vi "Vision Processing Boulder.vi"(4 "error in (no error)":errorcluster) -> ()   [LabVIEW 2015]
doc: "This VI runs in parallel to other tasks. It gets images from the camera, processes them for color or shape and uses commands or globals to affect the behavior of other subsystems."
uses:
  Framework/Robot Global Data.vi
  Support Code/ZMQ Library/socket_options.ctl
  Support Code/ZMQ Library/zeromq.lvlib
  Support Code/ZMQ Library/socket_type.ctl
  Support Code/ZMQ Library/zmq_context.lvclass
  Support Code/ZMQ Library/zmq_socket.lvclass
  Vision Published Globals.vi
  Intake/Implementation/Intake Published Globals.vi
panel:
  out "context out":refnum<class "zmq_context.lvclass">
  out "data 2":string
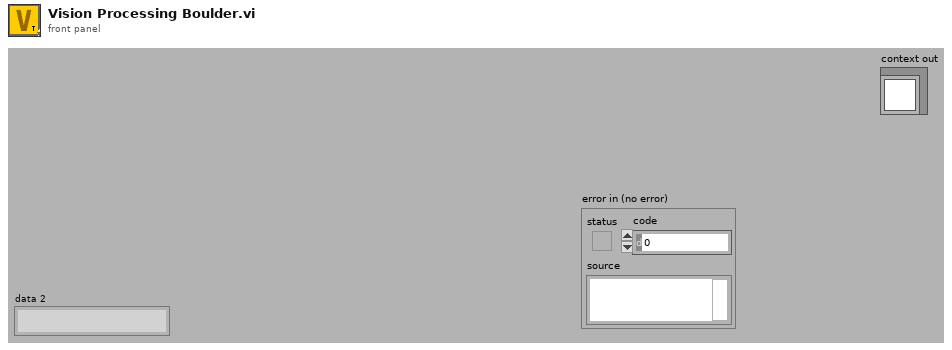
[diagram p1: front panel]
types:
  T1 = typedef "zeromq.lvlib/socket_options.ctl" = enum8{"NONE", "ZMQ_HWM", "<2>", "ZMQ_SWAP", "ZMQ_AFFINITY", "ZMQ_IDENTITY", "ZMQ_SUBSCRIBE", "ZMQ_UNSUBSCRIBE", "ZMQ_RATE", "ZMQ_RECOVERY_IVL", "ZMQ_MCAST_LOOP", "ZMQ_SNDBUF", "ZMQ_RCVBUF", "ZMQ_RCVMORE", "ZMQ_FD", "ZMQ_EVENTS", "ZMQ_TYPE", "ZMQ_LINGER", "ZMQ_RECONNECT_IVL", "ZMQ_BACKLOG", "ZMQ_RECOVERY_IVL_MSEC", "ZMQ_RECONNECT_IVL_MAX", "ZMQ_MAXMSGSIZE", "ZMQ_SNDHWM", "ZMQ_RCVHWM", "ZMQ_MULTICAST_HOPS", "<26>", "ZMQ_RCVTIMEO", "ZMQ_SNDTIMEO", "<29>", "<30>", "ZMQ_IPV4ONLY", "ZMQ_LAST_ENDPOINT", "ZMQ_ROUTER_MANDATORY", "ZMQ_TCP_KEEPALIVE", "ZMQ_TCP_KEEPALIVE_CNT", "ZMQ_TCP_KEEPALIVE_IDLE", "ZMQ_TCP_KEEPALIVE_INTVL", "ZMQ_TCP_ACCEPT_FILTER", "ZMQ_DELAY_ATTACH_ON_CONNECT", "ZMQ_XPUB_VERBOSE"}
  T2 = typedef "zeromq.lvlib/socket_type.ctl" = enum8{"ZMQ_PAIR", "ZMQ_PUB", "ZMQ_SUB", "ZMQ_REQ", "ZMQ_REP", "ZMQ_DEALER", "ZMQ_ROUTER", "ZMQ_PULL", "ZMQ_PUSH", "ZMQ_XPUB", "ZMQ_XSUB"}
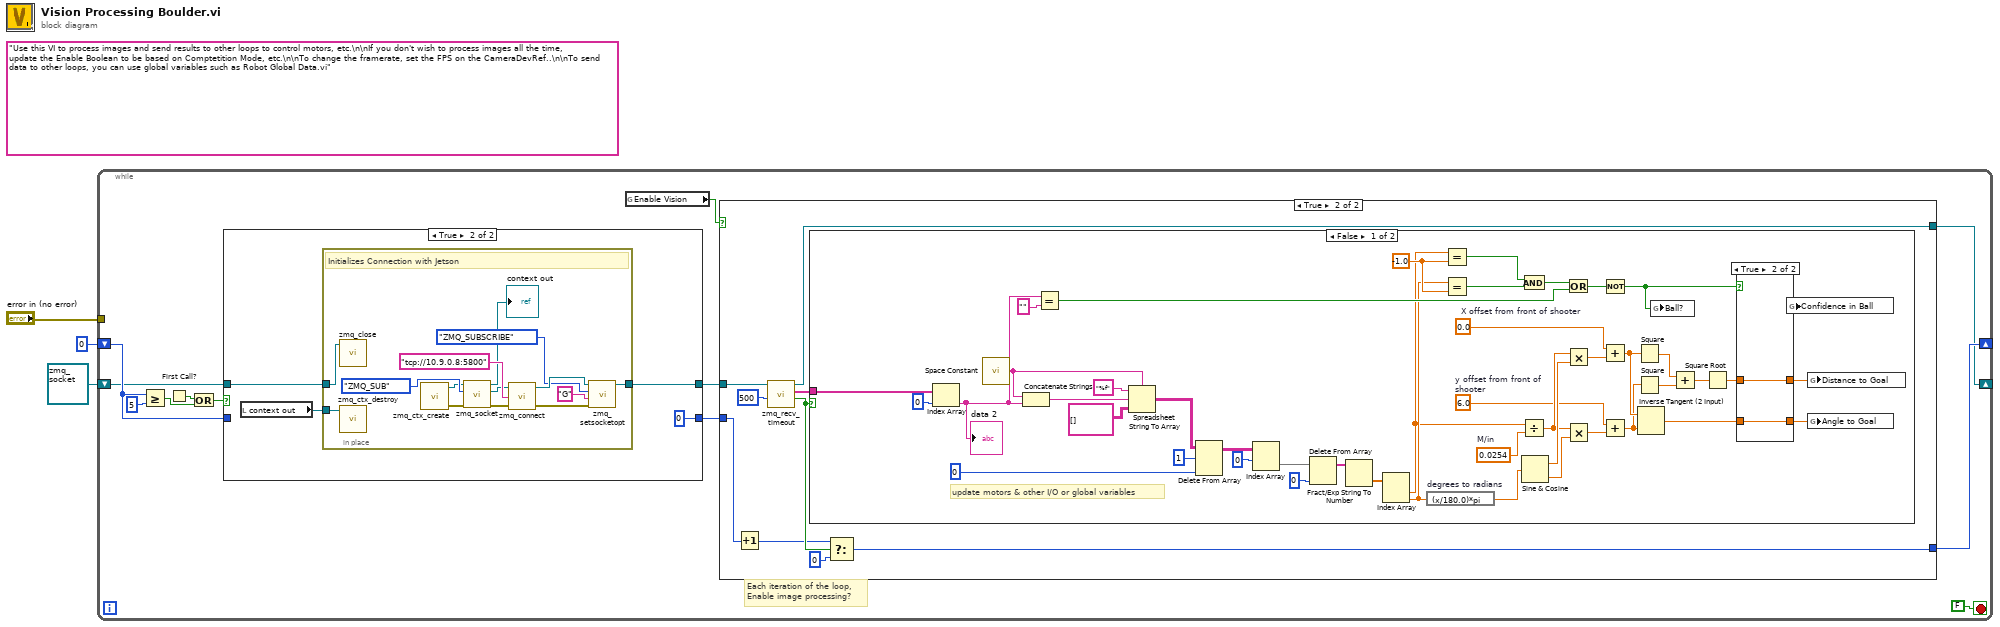
[diagram p0: block diagram]
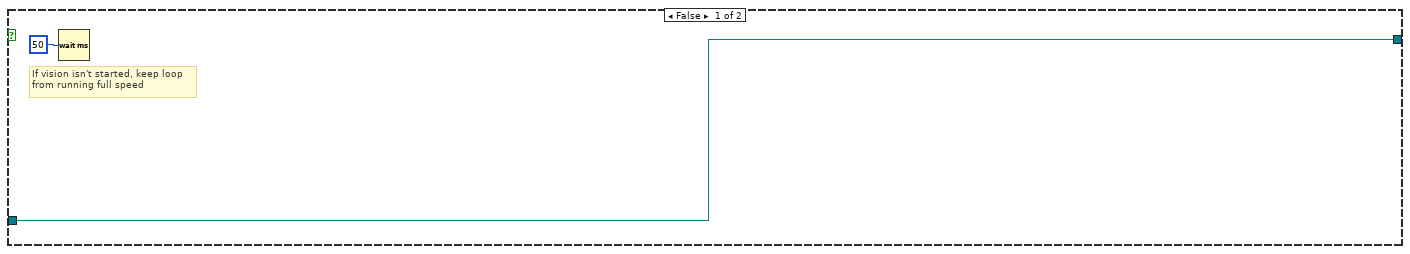
[diagram p3: hidden frame]
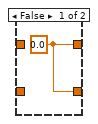
[diagram p4: hidden frame]
diagram:
  (unwired) "Use this VI to process images and send results to other loops to control motors, etc.\n\nIf you don't wish to process images all the time, update the Enable Boolean to be based on Comptetition Mode, etc.\n\nTo change the framerate, set the FPS on the CameraDevRef..\n\nTo send data to other loops, you can use global variables such as Robot Global Data.vi"
  n1 = while {
    tunnel: "error in (no error)" -> [_]
    shift-right: [w4] -> _
    shift-left: refnum<class "zmq_socket.lvclass"> refnum ("socket out") -> [w5]
    shift-right: [w13] -> _
    shift-left: 0 -> [w7]
    stop <- FALSE stop-if-true
    # "Each iteration of the loop,\nEnable image processing?"
    n2 = Greater Or Equal?(x=w7, y=5) -> (x >= y?=w11:bool)
    n3 = First Call?() -> (First Call?: T/F=w9:bool)
    n4 = Or(x=w9, y=w11) -> (x .or. y?=w10:bool)
    n5 = case shown="True" w10 {
      tunnel: [w17 0] -> w8
      tunnel: w7 -> [w17 _]
      tunnel: [w16 w20] -> w6
      tunnel: w5 -> [w16 w19]
      frame False {
      }
      frame True {
        n6 = local read "context out"() -> (w18:refnum<class "zmq_context.lvclass">)
        n7 = in-place {
          in-place-border: [w25] -> w20
          in-place-border: w19 -> [w22]
          in-place-border: w18 -> [w23]
          # "Initializes Connection with Jetson"
          n8 = call "zmq_close.vi"("socket"=w22) -> ()  [unwired: 4 in, 1 out]
          n9 = call "zmq_ctx_destroy.vi"("context in"=w23) -> ()  [unwired: 4 in, 1 out]
          n10 = call "zmq_ctx_create.vi"() -> ("error out"=w33:errorcluster, "context out"=w34:refnum<class "zmq_context.lvclass">)  [unwired: 4 in]
          n11 = call "zmq_socket.vi"("error in"=w33, "socket type"=socket_type."ZMQ_SUB", "context in"=w34) -> ("error out"=w30:errorcluster, "socket out"=w31:refnum<class "zmq_socket.lvclass">, "context out"=→"context out":refnum<class "zmq_context.lvclass">)  [unwired: 2 in]
          n12 = call "zmq_connect.vi"("error in"=w30, "endpoint"="tcp://10.9.0.8:5800" ("Endpoint"), "socket in"=w31) -> ("error out"=w27:errorcluster, "socket out"=w28:refnum<class "zmq_socket.lvclass">)  [unwired: 1 in]
          n13 = call "zmq_setsocketopt.vi"("error in"=w27, "value"="G", "option"=socket_options."ZMQ_SUBSCRIBE", "socket in"=w28) -> ("socket out"=w25:refnum<class "zmq_socket.lvclass">)  [unwired: 2 in, 1 out]
        }
      }
    }
    n14 = global read "Robot Global Data.vi" "Enable Vision"() -> (w14:bool)
    n15 = case shown="True" w14 {
      tunnel: w6 -> [w36 w45]
      tunnel: w8 -> [_ w41]
      tunnel: [_ w39] -> w13
      tunnel: [w36 w38] -> w4
      frame False {
        # "If vision isn't started, keep loop\nfrom running full speed"
        n16 = Wait (ms)(milliseconds to wait=u32 50) -> ()  [unwired: 1 out]
      }
      frame True {
        n17 = Increment(x=w41) -> (x+1=w42:i32)
        n18 = call "zmq_recv_timeout.vi"("timeout (ms)"=u32 500, "socket in"=w45) -> ("timeout?"=w43:bool, "parts"=w44:string[], "socket out"=w38:refnum<class "zmq_socket.lvclass">)  [unwired: 2 in, 1 out]
        n19 = case shown="False" w43 {
          tunnel: w44 -> [w52 _]
          frame False {
            w77 = 6.0  # y offset from front of shooter
            w78 = 0.0  # X offset from front of shooter
            w90 = 0.0254  # M/in
            w71 = -1.0 ("y")
            # "update motors & other I/O or global variables"
            n20 = Index Array(array=w52, index=0) -> (element=w50:string)
            "data 2" <- w50
            n21 = call <vilib>:"Space Constant.vi"() -> ("String"=w59:string)
            n22 = Concatenate Strings(w59, w50) -> (w60:string)
            n23 = Equal?(x=w50, y="") -> (x = y?=w75:bool)
            n24 = Spreadsheet String To Array(delimiter (Tab)=w59, format string="%f", spreadsheet string=w60, array type (2D Dbl)=string[][] [] ("Array")) -> (array=w61:string[][])
            n25 = Delete From Array(array=w61, length=1, index (col)=0 ("disabled index (col)")) -> (array with subset deleted=w58:string[][])  [unwired: 1 in, 1 out]
            n26 = Index Array(array=w58, index (row)=0) -> (element=w55:string[])  [unwired: 1 in]
            n27 = Delete From Array(array=w55, index=0) -> (array with subset deleted=w54:string[])  [unwired: 1 in, 1 out]
            n28 = Fract/Exp String To Number(string=w54) -> (number=w51:dbl[])  [unwired: 4 out]
            n29 = Index Array(array=w51) -> (element #1=w66:dbl, element #2=w67:dbl)  [unwired: 2 in]
            n30 = expression code="(x/180.0)*pi" "degrees to radians"(w67) -> (w89:dbl)
            n31 = Equal?(x=w66, y=w71) -> (x = y?=w69:bool)
            n32 = Equal?(x=w67, y=w71) -> (x = y?=w70:bool)
            n33 = And(x=w69, y=w70) -> (x .and. y?=w68:bool)
            n34 = Divide(x=w66, y=w90) -> (x/y=w85:dbl)
            n35 = Sine & Cosine(0:w89) -> (1:w88:dbl, 2:w86:dbl)
            n36 = Or(x=w68, y=w75) -> (x .or. y?=w74:bool)
            n37 = Multiply(x=w85, y=w88) -> (x*y=w87:dbl)
            n38 = Multiply(x=w85, y=w86) -> (x*y=w84:dbl)
            n39 = Not(x=w74) -> (.not. x?=w47:bool)
            n40 = Add(x=w78, y=w87) -> (x+y=w80:dbl)
            n41 = Add(x=w77, y=w84) -> (x+y=w79:dbl)
            n42 = Square(x=w80) -> (x^2=w83:dbl)
            n43 = Square(x=w79) -> (x^2=w82:dbl)
            n44 = Inverse Tangent (2 Input)(1:w79, 2:w80) -> (0:w73:dbl)
            n45 = global write "Intake Published Globals.vi" "Ball?"(w47) -> ()
            n46 = Add(x=w83, y=w82) -> (x+y=w81:dbl)
            n47 = Square Root(x=w81) -> (sqrt(x)=w72:dbl)
            n48 = case shown="True" w47 {
              tunnel: [w91 w93] -> w49
              tunnel: w73 -> [_ w93]
              tunnel: [w91 w92] -> w48
              tunnel: w72 -> [_ w92]
              frame False {
                w91 = 0.0
              }
              frame True {
              }
            }
            n49 = global read "Vision Published Globals.vi" "Confidence in Ball"() -> ()  [unwired: 1 in]
            n50 = global write "Vision Published Globals.vi" "Distance to Goal"(w48) -> ()
            n51 = global write "Vision Published Globals.vi" "Angle to Goal"(w49) -> ()
          }
          frame True {
          }
        }
        n52 = Select(t=w42, s=w43, f=0) -> (s? t:f=w39:i32)
      }
    }
  }
